vi "database_connection_write_dev.vi"(5 "ODBC data source name":string="amrc_monitoring", 6 "error in (no error)":errorcluster, 7 "G1?":u32, 8 "current time":timestamp, 9 "data 2":dbl[](array[numeric]), 10 "Machine Data":T1={"Zload"="", "Yload"="", "Xload"="", "path_position"="", "Fovr"="", "SspeedOvr"="", "Program Name"="", "Program status"="", "Block of code being executed"="", "Line of code"="", "Machine availability"="", "Emergency status"="", "Controller mode"="", "Tool_id"="UNAVAILABLE"}, 11 "Machine type":string) -> (3 "error out":errorcluster)   [LabVIEW 2017]
uses:
  <vilib>/addons/database/Connection.llb/DB Tools Open Connec (Path).vi
  <vilib>/addons/database/Connection.llb/Conn Execute.vi
  <vilib>/addons/database/Recordset.llb/Rec Destroy - Connection.vi
  <vilib>/regexp/Match Regular Expression.xnode
  <vilib>/addons/database/NI_Database_API.lvlib
panel:
  out "string":string="(timestamp,machine_status,g1,tool_id,force_acc_raw_data,spike_raw_data,spindle_load,spindle_speed,feed_rate,I,J,K,X,Y,Z,position_A,position_B ,Xload,Yload,Zload,Aload,Bload,program_number,accel_x_rms,accel_y_rms,accel_z_rms,force_x_rms,force_y_rms,force_z_rms,axial_force_rms, torque_rms,bending_x_rms,bending_y_rms,estop,block_code,fovr,sspeedovr,program_name,line) VALUES ("
  out "data 3":dbl[](array[numeric])
  out "path_position":string
  out "x = y?":bool
  out "submatch 1":string
  out "after match 3":string
  out "empty? 2":bool
  out "after match 2":string
  out "resulting string 4":string
  out "Xload":string
  out "concatenated string 6":string
  out "resulting string 3":string
  out "concatenated string 2":string
  out "resulting string 2":string
  out "ODBC data source name 2":string="amrc_monitoring"
  out "resulting string":string
  out "size(s)":i32
  out "concatenated string 5":string
  out "concatenated string 3":string
  out "concatenated string":string
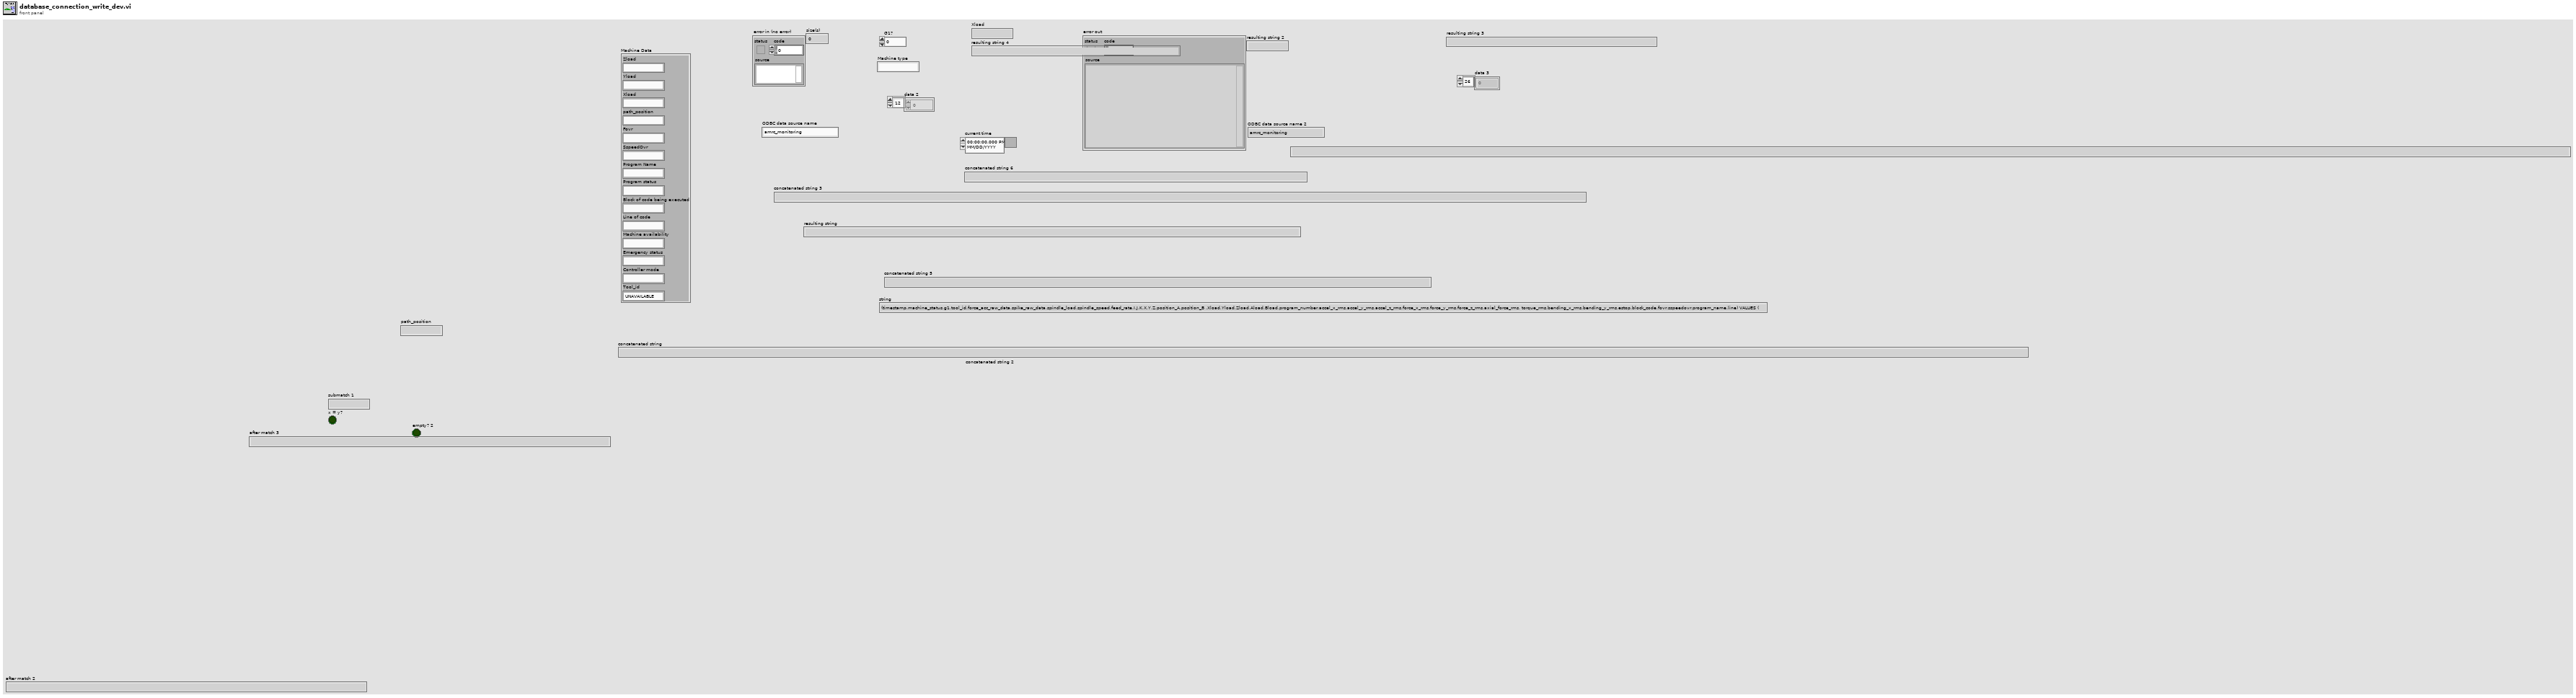
[diagram p1: front panel]
types:
  T1 = cluster{"Zload":string, "Yload":string, "Xload":string, "path_position":string, "Fovr":string, "SspeedOvr":string, "Program Name":string, "Program status":string, "Block of code being executed":string, "Line of code":string, "Machine availability":string, "Emergency status":string, "Controller mode":string, "Tool_id":string}
  T2 = typedef "NI_Database_API.lvlib/Conn ObjectReference.ctl" = refnum<k1>
  T3 = typedef "NI_Database_API.lvlib/Rec ObjectReference.ctl" = refnum<k1>
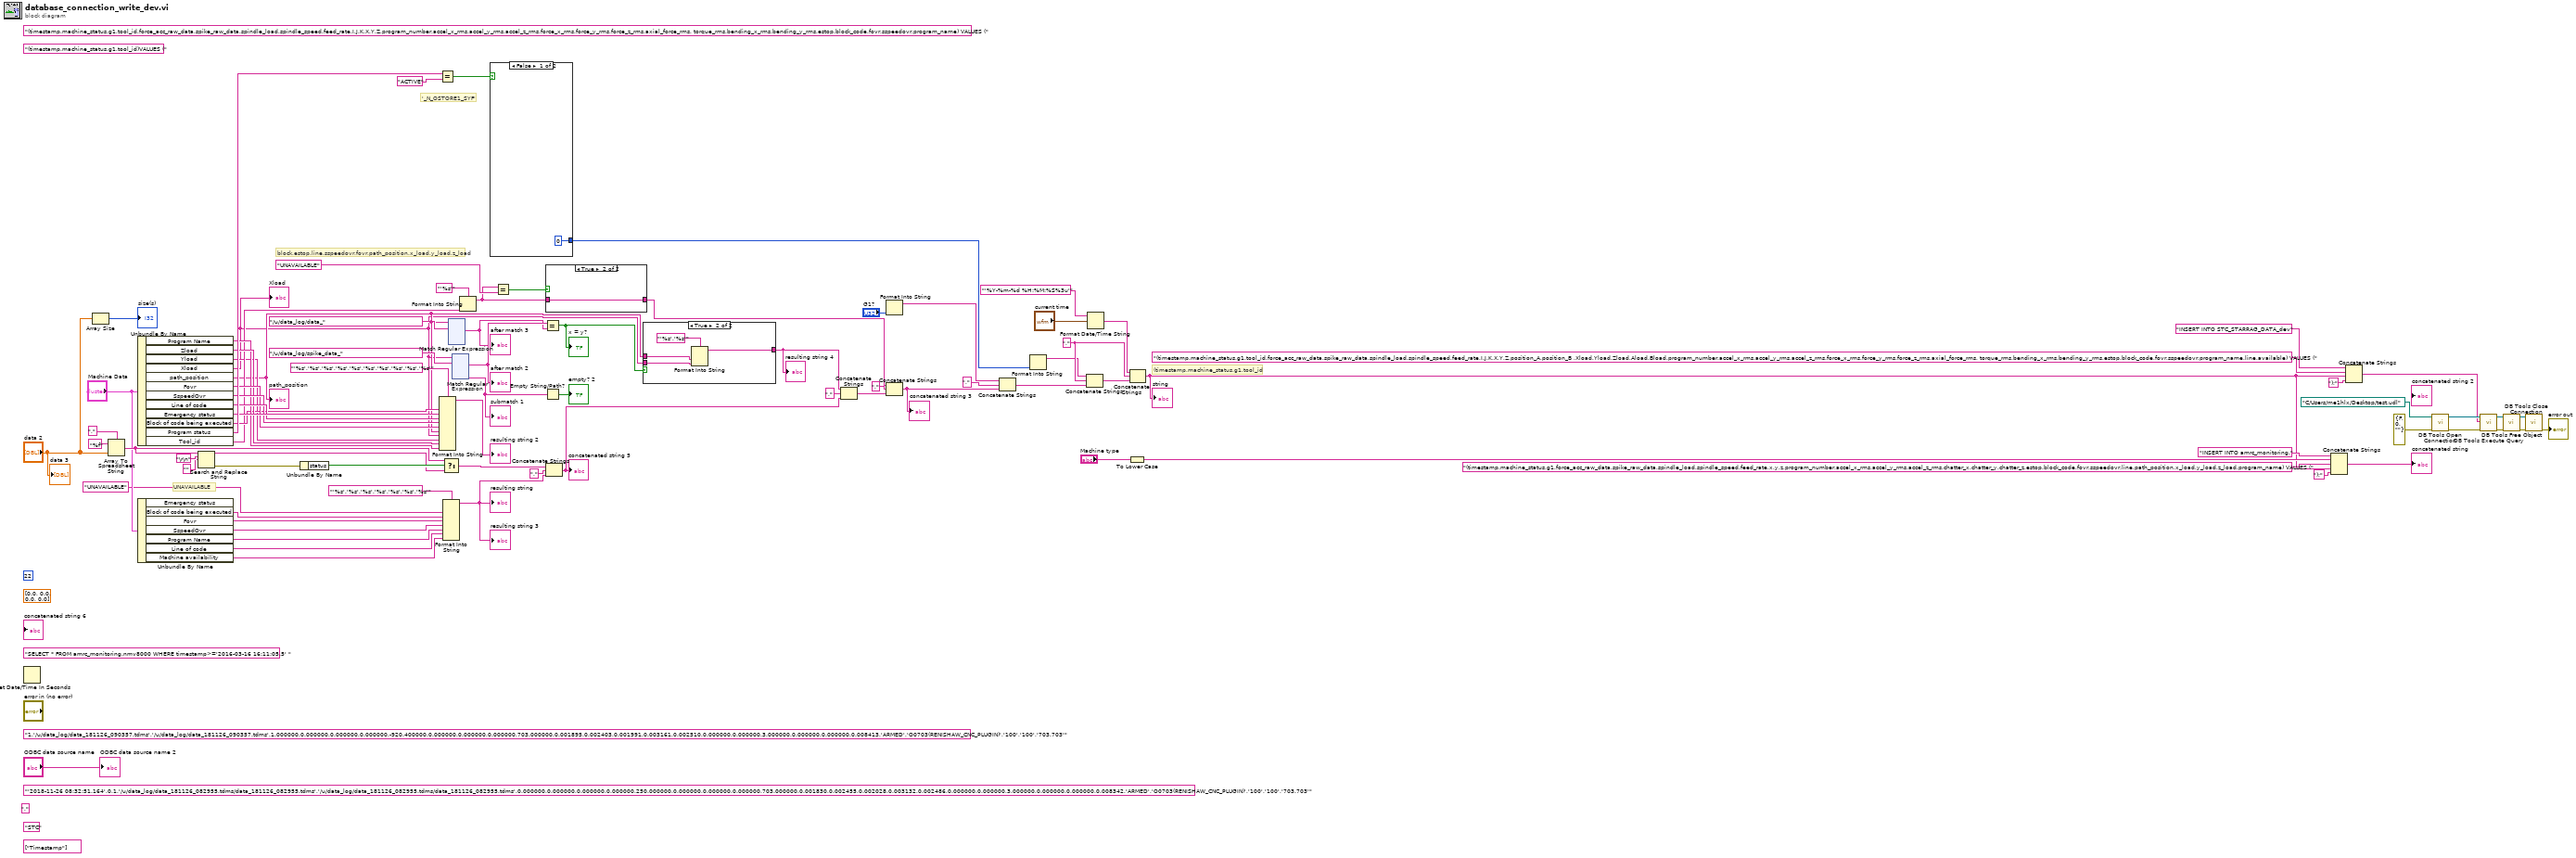
[diagram p0: block diagram]
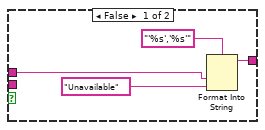
[diagram p2: hidden frame]
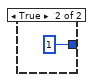
[diagram p4: hidden frame]
diagram:
  (unwired) "(timestamp,machine_status,g1,tool_id,force_acc_raw_data,spike_raw_data,spindle_load,spindle_speed,feed_rate,I,J,K,X,Y,Z,program_number,accel_x_rms,accel_y_rms,accel_z_rms,force_x_rms,force_y_rms,force_z_rms,axial_force_rms, torque_rms,bending_x_rms,bending_y_rms,estop,block_code,fovr,sspeedovr,program_name) VALUES (" ("string")
  (unwired) "(timestamp,machine_status,g1,tool_id)VALUES (" ("string")
  (unwired) dbl[] [0.0, 0.0, 0.0, 0.0]
  (unwired) "1,'/u/data_log/data_181126_090357.tdms','/u/data_log/data_181126_090357.tdms',1.000000,0.000000,0.000000,0.000000,-920.400000,0.000000,0.000000,0.000000,703.000000,0.001895,0.002403,0.001991,0.003161,0.002510,0.000000,0.000000,3.000000,0.000000,0.000000,0.008413,'ARMED','O0703(RENISHAW_CNC_PLUGIN)','100','100','703.703'" ("concatenated string 4")
  (unwired) "'2018-11-26 08:32:51.164',0,1,'/u/data_log/data_181126_082955.tdms/data_181126_082955.tdms','/u/data_log/data_181126_082955.tdms/data_181126_082955.tdms',0.000000,0.000000,0.000000,0.000000,250.000000,0.000000,0.000000,0.000000,703.000000,0.001830,0.002455,0.002028,0.003132,0.002486,0.000000,0.000000,3.000000,0.000000,0.000000,0.008342,'ARMED','O0703(RENISHAW_CNC_PLUGIN)','100','100','703.703'" ("concatenated string 2")
  (unwired) 22
  (unwired) "," ("string")
  (unwired) string[] ["Timestamp"]
  (unwired) "STC"
  w47 = "," ("string")
  (unwired) "SELECT * FROM amrc_monitoring.nmv8000 WHERE timestamp>='2016-03-16 16:11:05.5' " ("SQL query")
  # "(timestamp,machine_status,g1,tool_id"
  # "'_N_OSTORE1_SYF'"
  # "UNAVAILABLE"
  # "block,estop,line,sspeedovr,fovr,path_position,x_load,y_load,z_load"
  n1 = Get Date/Time In Seconds() -> ()  [unwired: 1 out]
  n2 = Array Size(array="data 2") -> (size(s)=→"size(s)":i32)
  n3 = Array To Spreadsheet String(delimiter (Tab)=",", array="data 2", 3:"%f" ("format string")) -> (spreadsheet string=w73:string)
  n4 = Unbundle By Name("Machine Data") -> ("Program Name"=w60:string, "Zload"=w64:string, "Yload"=w26:string, "Xload"=w7:string, "path_position"=w8:string, "Fovr"=w65:string, "SspeedOvr"=w66:string, "Line of code"=w67:string, "Emergency status"=w68:string, "Block of code being executed"=w58:string, "Program status"=w86:string, "Tool_id"=w52:string)
  "Xload" <- w7
  "path_position" <- w8
  n5 = Unbundle By Name("Machine Data") -> ("Block of code being executed"=w33:string, "Fovr"=w32:string, "SspeedOvr"=w31:string, "Program Name"=w30:string, "Line of code"=w5:string, "Machine availability"=w2:string)  [unwired: 1 out]
  n6 = Search and Replace String(input string=w73, search string="\r\n", replace string="" ("replace string (\"\")")) -> (result string=w74:string, error out=w76:errorcluster)  [unwired: 5 in, 2 out]
  n7 = Unbundle By Name(w76) -> ("status"=w75:bool)
  n8 = Format Into String(format string="'%s','%s','%s','%s','%s','%s','%s','%s','%s','%s'", w58, w68, w67, w66, w65, w8, w7, w26, w64, w60) -> (resulting string=→"resulting string 2":string)  [unwired: 2 in, 1 out]
  n9 = Equal?(x=w86, y="ACTIVE") -> (x = y?=w84:bool)
  n10 = Select(t=w73, s=w75, f=w74) -> (s? t:f=w61:string)
  n11 = Format Into String(format string="'%s','%s','%s','%s','%s','%s','%s'", "UNAVAILABLE" ("format string"), w33, w32, w31, w30, w5, w2) -> (resulting string=w25:string)  [unwired: 2 in, 1 out]
  "resulting string" <- w25
  "resulting string 3" <- w25
  n12 = xnode "Match Regular Expression"("input string"=w8, "regular expression"="/u/data_log/data_") -> ("after match"=w10:string)  [unwired: 4 in, 5 out]
  "after match 3" <- w10
  n13 = xnode "Match Regular Expression"("input string"=w7, "regular expression"="/u/data_log/spike_data_") -> ("after match"=w11:string, "submatch 1"=w12:string)  [unwired: 4 in, 4 out]
  "after match 2" <- w11
  "submatch 1" <- w12
  n14 = Format Into String(format string="'%s'", w52) -> (resulting string=w51:string)  [unwired: 2 in, 1 out]
  n15 = case shown="False" w84 {
    tunnel: [0 1] -> w22
    frame False {
    }
    frame True {
    }
  }
  n16 = Equal?(x=w51, y="UNAVAILABLE") -> (x = y?=w83:bool)
  n17 = Equal?(x=w11, y=w10) -> (x = y?=w9:bool)
  "x = y?" <- w9
  n18 = Empty String/Path?(string/path=w12) -> (empty?=→"empty? 2":bool)
  n19 = case shown="True" w83 {
    tunnel: w51 -> [w91 w92]
    tunnel: [w91 w92] -> w3
    frame False {
    }
    frame True {
    }
  }
  n20 = Concatenate Strings(w61, "," ("string"), w25) -> (w19:string)
  "concatenated string 5" <- w19
  n21 = case shown="True" w9 {
    tunnel: w8 -> [w95 w97]
    tunnel: w7 -> [_ w100]
    tunnel: [w94 w98] -> w6
    frame False {
      n22 = Format Into String(format string="'%s','%s'", w95, "Unavailable" ("Tool_id")) -> (resulting string=w94:string)  [unwired: 2 in, 1 out]
    }
    frame True {
      n23 = Format Into String(format string="'%s','%s'", w97, w100) -> (resulting string=w98:string)  [unwired: 2 in, 1 out]
    }
  }
  "resulting string 4" <- w6
  n24 = Concatenate Strings(w6, "," ("string"), w19) -> (w17:string)
  n25 = Format Into String("G1?") -> (resulting string=w45:string)  [unwired: 3 in, 1 out]
  n26 = Concatenate Strings(w3, "," ("string"), w17) -> (w23:string)
  "concatenated string 3" <- w23
  n27 = Concatenate Strings(w45, "," ("string"), w23) -> (w24:string)
  n28 = Format Into String(w22) -> (resulting string=w46:string)  [unwired: 3 in, 1 out]
  n29 = Concatenate Strings(w46, w47, w24) -> (w79:string)
  n30 = Format Date/Time String(time format string (%c)="'%Y-%m-%d %H:%M:%S%3u'", seconds (now)="current time") -> (date/time string=w48:string)  [unwired: 1 in]
  n31 = To Lower Case(string="Machine type") -> (all lower case string=w70:string)
  n32 = Concatenate Strings(w48, w47, w79) -> (w4:string)
  "string" <- w4
  n33 = Concatenate Strings("INSERT INTO amrc_monitoring." ("string"), w70, "(timestamp,machine_status,g1,force_acc_raw_data,spike_raw_data,spindle_load,spindle_speed,feed_rate,x,y,z,program_number,accel_x_rms,accel_y_rms,accel_z_rms,chatter_x,chatter_y,chatter_z,estop,block_code,fovr,sspeedovr,line,path_position,x_load,y_load,z_load,program_name) VALUES (" ("string"), w4, ");" ("string")) -> (→"concatenated string":string)
  n34 = Concatenate Strings("INSERT INTO STC_STARRAG_DATA_dev" ("string"), "(timestamp,machine_status,g1,tool_id,force_acc_raw_data,spike_raw_data,spindle_load,spindle_speed,feed_rate,I,J,K,X,Y,Z,position_A,position_B ,Xload,Yload,Zload,Aload,Bload,program_number,accel_x_rms,accel_y_rms,accel_z_rms,force_x_rms,force_y_rms,force_z_rms,axial_force_rms, torque_rms,bending_x_rms,bending_y_rms,estop,block_code,fovr,sspeedovr,program_name,line,available) VALUES (" ("string"), w4, ");" ("string")) -> (w1:string)
  n35 = call-poly <vilib>:"DB Tools Open Connection.vi"("error in (no error)"=errorcluster {"status"=FALSE, "code"=0, "source"=""}, "connection information"=path "C:/Users/me1hlx/Desktop/test.udl") -> ("error out"=w44:errorcluster, "connection reference"=w38:T2)  [unwired: 6 in]
  n36 = call-poly <vilib>:"DB Tools Execute Query.vi"("error in (no error)"=w44, "SQL query"=w1, "connection reference"=w38) -> ("error out"=w41:errorcluster, "recordset reference"=w42:T3)  [unwired: 5 in]
  n37 = call-poly <vilib>:"DB Tools Free Object.vi"("error in (no error)"=w41, "recordset reference"=w42) -> ("error out"=w39:errorcluster, "connection reference"=w40:T2)  [unwired: 8 in]
  n38 = call <vilib>:"DB Tools Close Connection.vi"("error in (no error)"=w39, "connection reference"=w40) -> ("error out"=→"error out":errorcluster)  [unwired: 5 in]
  "ODBC data source name 2" <- "ODBC data source name"
  "data 3" <- "data 2"
